vi "Analyze GB - Detail.vi"(8 "Integer Tolerance":dbl=0.1, 10 "Find Integer Rep?":bool, 11 "Grain Boundary Definition":T1={"Grain 1 Orientation"=[1.0, 1.0, 1.0], "Grain 2 Orientation"=[1.0, 1.0, 1.0], "Twist Angle (Deg)"=60.0, "Translation Vector"=[0.0, 0.0, 0.0]}) -> (0 "STEM Viewing Angles":dbl[][](array[numeric]), 1 "Misorientation":T3={"Misorientation Angle"=0.0, "Misorientation Axis, o"=[1.0, 1.0, 1.0], "Misorientation Matrix"=[]}, 2 "Grain 2 Integers":dbl[](array[numeric])=[1.0, 1.0, 1.0], 3 "Grain 1 Integers":dbl[](array[numeric])=[1.0, 1.0, 1.0], 4 "Tilt Angle (Deg)":dbl, 5 "Suggested view direction":dbl[](array[numeric])=[1.0, 1.0, 1.0], 6 "GB Name":string, 7 "STEM Viewable?":bool)   [LabVIEW 2010]
uses:
  <vilib>/Analysis/Matrix/Datatypes/RealMatrix.ctl
  <vilib>/Analysis/baseanly.llb/Real A x B.vi
  <vilib>/Analysis/_algsub.llb/Real Matrix Trace.vi
  <vilib>/Analysis/NI_AALPro.lvlib
  <vilib>/Analysis/NI_AALBase.lvlib
  <vilib>/Analysis/Matrix/NI_Matrix.lvlib
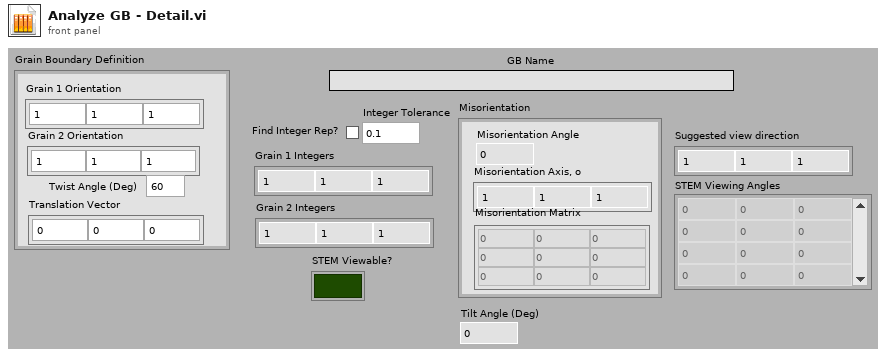
[diagram p1: front panel]
types:
  T1 = cluster{"Grain 1 Orientation":dbl[], "Grain 2 Orientation":dbl[], "Twist Angle (Deg)":dbl, "Translation Vector":dbl[]}
  T2 = typedef "NI_Matrix.lvlib/RealMatrix.ctl" = dbl[][]
  T3 = cluster{"Misorientation Angle":dbl, "Misorientation Axis, o":dbl[], "Misorientation Matrix":T2}
  T4 = cluster{"Grain 1 Orientation":dbl[], "Grain 2 Orientation":dbl[], "Twist Angle (Deg)":dbl}
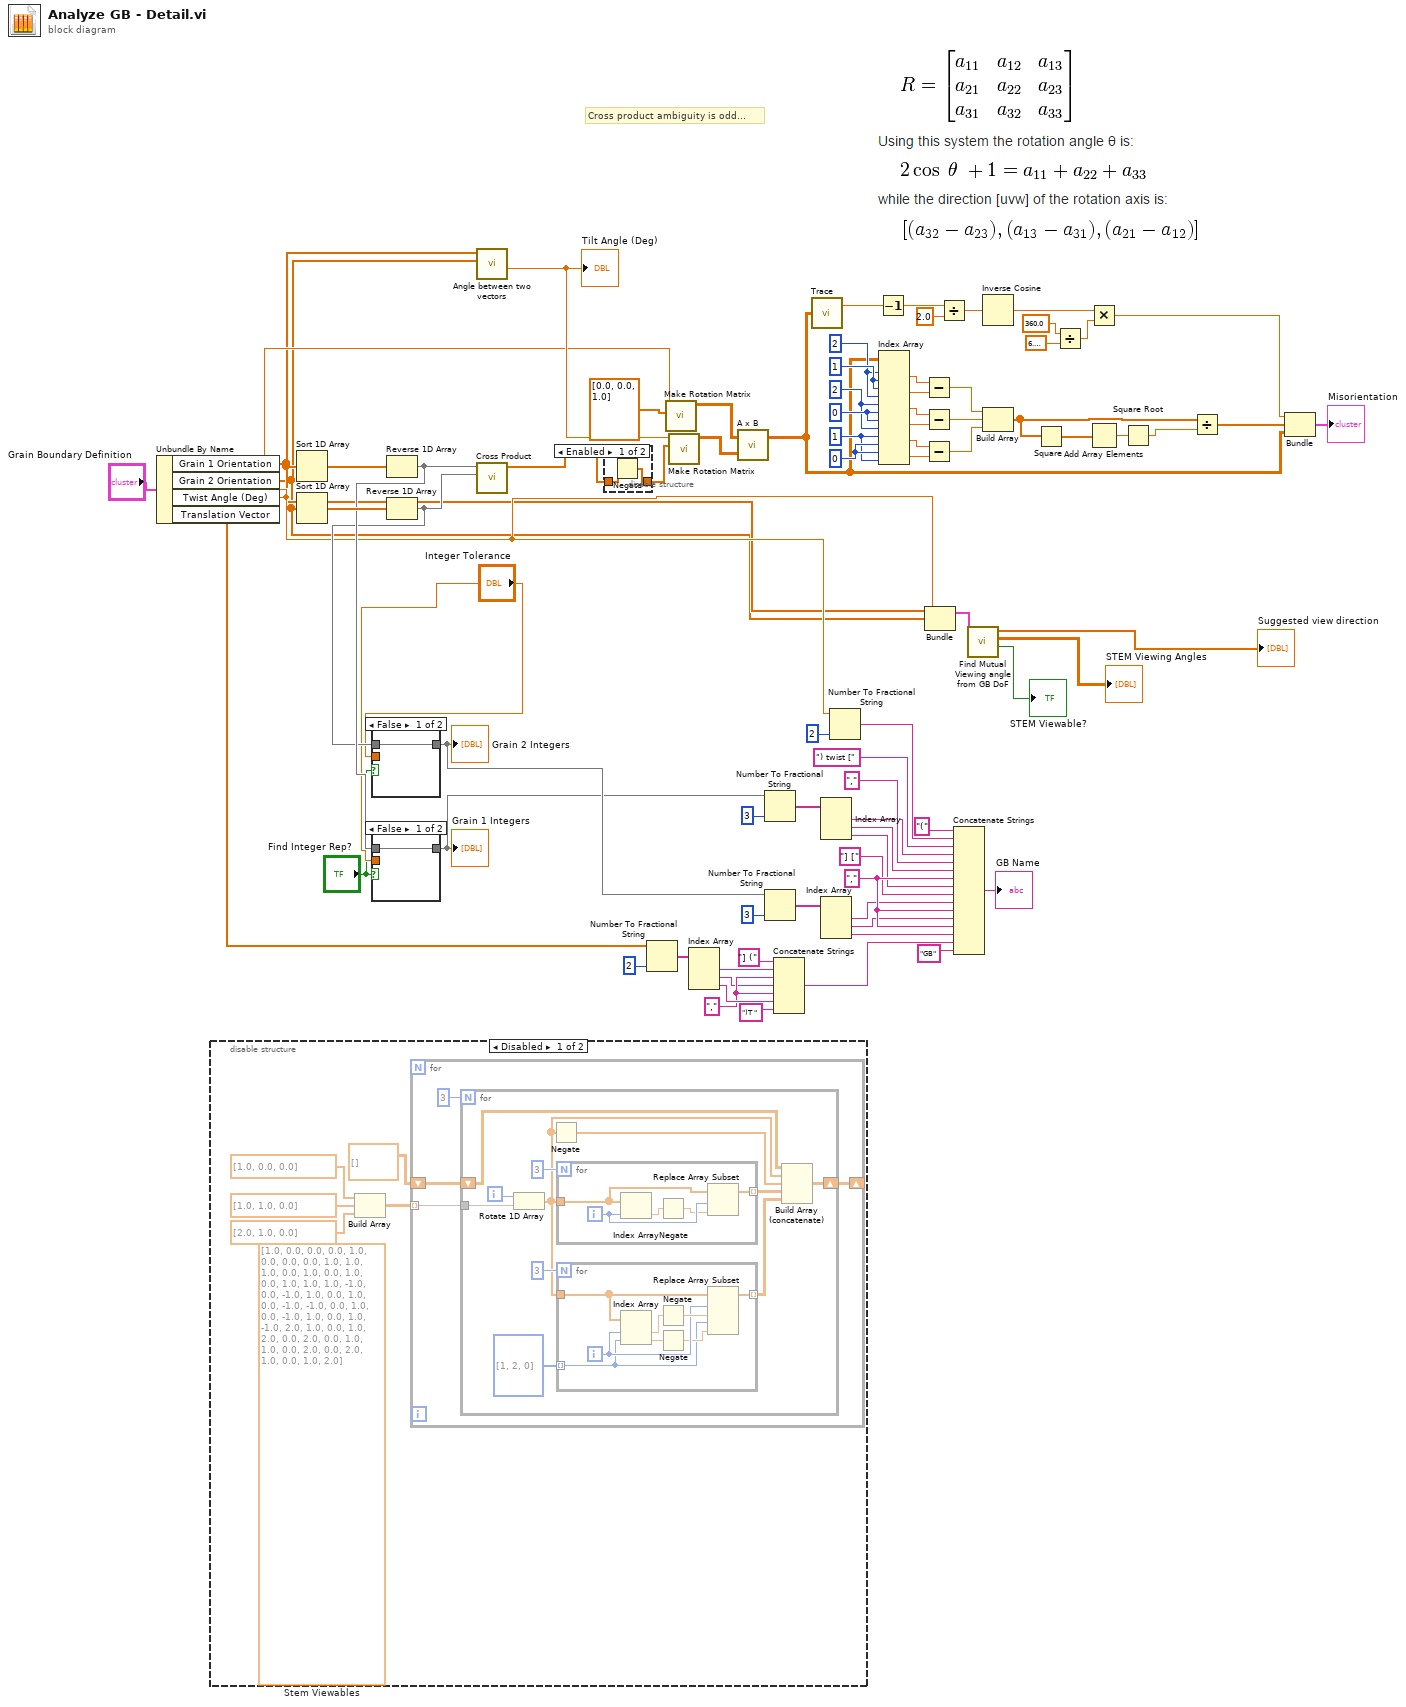
[diagram p0: block diagram]
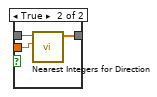
[diagram p3: hidden frame]
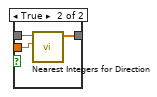
[diagram p4: hidden frame]
diagram:
  w38 = "," ("string")
  w31 = "," ("string")
  w63 = 0 ("index (row)")
  w62 = 1 ("index (row)")
  w65 = 0 ("disabled index (col)")
  w64 = 2 ("index (row)")
  w67 = 1 ("disabled index (col)")
  w66 = 2 ("index (row)")
  # "Cross product ambiguity is odd..."
  n1 = Unbundle By Name("Grain Boundary Definition") -> ("Grain 1 Orientation"=w3:dbl[], "Grain 2 Orientation"=w2:dbl[], "Twist Angle (Deg)"=w8:dbl, "Translation Vector"=w9:dbl[])
  n2 = disable-structure shown="Disabled" {
    frame Disabled {
      (unwired) dbl[][] [[1.0, 0.0, 0.0], [0.0, 1.0, 0.0], [0.0, 0.0, 1.0], [1.0, 1.0, 0.0], [1.0, 0.0, 1.0], [0.0, 1.0, 1.0], [1.0, -1.0, 0.0], [-1.0, 1.0, 0.0], [1.0, 0.0, -1.0], [-1.0, 0.0, 1.0], [0.0, -1.0, 1.0], [0.0, 1.0, -1.0], [2.0, 1.0, 0.0], [1.0, 2.0, 0.0], [2.0, 0.0, 1.0], [1.0, 0.0, 2.0], [0.0, 2.0, 1.0], [0.0, 1.0, 2.0]]  # Stem Viewables
      n3 = Build Array(dbl[] [1.0, 0.0, 0.0] ("Grain 1 Orientation 2"), dbl[] [1.0, 1.0, 0.0] ("Grain 1 Orientation 2"), dbl[] [2.0, 1.0, 0.0] ("Grain 1 Orientation 2")) -> (w84:dbl[][])
      n4 = for {
        tunnel: w84 -> [w90] mode=indexing
        shift-right: [w89] -> _
        shift-left: dbl[][] [] -> [w88]
        n5 = for {
          N: 3 -> [_]
          tunnel: w90 -> [w102]
          shift-right: [w96] -> w89
          shift-left: w88 -> [w95]
          i -> [w101]
          n6 = Rotate 1D Array(1:w102, 2:w101) -> (0:w92:dbl[])
          n7 = Negate(x=w92) -> (-x=w93:dbl[])
          n8 = for {
            N: 3 -> [_]
            tunnel: w92 -> [w114]
            tunnel: [w111] -> w98 mode=indexing
            i -> [w113]
            n9 = Index Array(array=w114, index=w113) -> (element=w115:dbl)
            n10 = Negate(x=w115) -> (-x=w112:dbl)
            n11 = Replace Array Subset(array=w114, new element=w112, index=w113) -> (w111:dbl[])
          }
          n12 = for {
            N: 3 -> [_]
            tunnel: w92 -> [w109]
            tunnel: [w106] -> w97 mode=indexing
            tunnel: i32[] [1, 2, 0] -> [w103] mode=indexing
            i -> [w105]
            n13 = Index Array(array=w109, index #1=w105, index #2=w103) -> (element #1=w110:dbl, element #2=w107:dbl)
            n14 = Negate(x=w110) -> (-x=w108:dbl)
            n15 = Negate(x=w107) -> (-x=w104:dbl)
            n16 = Replace Array Subset(array=w109, new element #1=w108, index #1=w105, new element #2=w104, index #2=w103) -> (w106:dbl[])
          }
          n17 = Build Array (concatenate)(w95, w92, w93, w98, w97) -> (w96:dbl[][])
        }
      }
    }
    frame Enabled {
    }
  }
  n18 = Sort 1D Array(array=w3) -> (sorted array=w82:dbl[])
  n19 = Sort 1D Array(array=w2) -> (sorted array=w81:dbl[])
  n20 = Reverse 1D Array(array=w82) -> (reversed array=w56:dbl[])
  n21 = case shown="False" "Find Integer Rep?" {
    tunnel: [w116 w119] -> w10
    tunnel: w56 -> [w116 w118]
    tunnel: "Integer Tolerance" -> [_ w117]
    frame False {
    }
    frame True {
      n22 = call "Nearest Integers for Direction.vi"("Tolerance"=w117, "Direction"=w118) -> ("Nearest Integer Directions"=w119:dbl[])  [unwired: 8 in, 1 out]
    }
  }
  "Grain 1 Integers" <- w10
  n23 = Reverse 1D Array(array=w81) -> (reversed array=w51:dbl[])
  n24 = case shown="False" "Find Integer Rep?" {
    tunnel: [w120 w123] -> w11
    tunnel: w51 -> [w120 w122]
    tunnel: "Integer Tolerance" -> [_ w121]
    frame False {
    }
    frame True {
      n25 = call "Nearest Integers for Direction.vi"("Tolerance"=w121, "Direction"=w122) -> ("Nearest Integer Directions"=w123:dbl[])  [unwired: 8 in, 1 out]
    }
  }
  "Grain 2 Integers" <- w11
  n26 = call "Angle between two vectors.vi"("Vector 2"=w2, "Vector 1"=w3) -> ("Angle (Degrees)"=w72:dbl)  [unwired: 7 in, 2 out]
  "Tilt Angle (Deg)" <- w72
  n27 = call <vilib>:"Cross Product.vi"("B Vector"=w51, "A Vector"=w56) -> ("Cross Product"=w43:dbl[])  [unwired: 8 in, 1 out]
  n28 = disable-structure shown="Enabled" {
    disable-tunnel: w43 -> [w125 w126]
    disable-tunnel: [w124 w126] -> w42
    frame Enabled {
      n29 = Negate(x=w125) -> (-x=w124:dbl[])
    }
    frame Disabled {
    }
  }
  n30 = Number To Fractional String(number=w9, precision (6)=i16 2) -> (F-format string=w34:string[])  [unwired: 2 in]
  n31 = call "Make Rotation Matrix.vi"("Rotation Axis"=dbl[] [0.0, 0.0, 1.0], "Rotation Angle (Degree)"=w8) -> ("Rotation Matrix"=w44:T2)  [unwired: 9 in]
  n32 = call "Make Rotation Matrix.vi"("Rotation Axis"=w42, "Rotation Angle (Degree)"=w72) -> ("Rotation Matrix"=w45:T2)  [unwired: 9 in]
  n33 = Index Array(array=w34) -> (element #1=w35:string, element #2=w37:string, element #3=w39:string)  [unwired: 3 in]
  n34 = call-poly <vilib>:"A x B.vi"("B"=w45, "A"=w44) -> ("A x B"=w47:T2)  [unwired: 1 out]
  n35 = Number To Fractional String(number=w10, precision (6)=i16 3) -> (F-format string=w18:string[])  [unwired: 2 in]
  n36 = Number To Fractional String(number=w11, precision (6)=i16 3) -> (F-format string=w16:string[])  [unwired: 2 in]
  n37 = Concatenate Strings("] (" ("string"), w35, w38, w37, w38, w39, ")T " ("string")) -> (w15:string)
  n38 = call-poly <vilib>:"Trace.vi"("Input Matrix"=w47) -> ("trace"=w80:dbl)  [unwired: 1 out]
  n39 = Index Array(array=w18) -> (element #1=w24:string, element #2=w26:string, element #3=w27:string)  [unwired: 3 in]
  n40 = Index Array(array=w16) -> (element #1=w29:string, element #2=w30:string, element #3=w32:string)  [unwired: 3 in]
  n41 = Number To Fractional String(number=w8, precision (6)=i16 2) -> (F-format string=w22:string)  [unwired: 2 in]
  n42 = Decrement(x=w80) -> (x-1=w79:dbl)
  n43 = Index Array(array=w47, index (row) #1=w66, index (col) #1=w67, index (row) #2=w67, index (col) #2=w66, index (row) #3=w64, index (col) #3=w65, index (row) #4=w65, index (col) #4=w64, index (row) #5=w62, index (col) #5=w63, index (row) #6=w63, index (col) #6=w62) -> (element #1=w71:dbl, element #2=w70:dbl, element #3=w69:dbl, element #4=w68:dbl, element #5=w61:dbl, element #6=w60:dbl)
  n44 = Subtract(x=w71, y=w70) -> (x-y=w59:dbl)
  n45 = Subtract(x=w69, y=w68) -> (x-y=w58:dbl)
  n46 = Subtract(x=w61, y=w60) -> (x-y=w57:dbl)
  n47 = Bundle("Grain 1 Orientation"=w3, "Grain 2 Orientation"=w2, "Twist Angle (Deg)"=w8) -> (w7:T4)  [unwired: 1 in]
  n48 = Divide(x=w79, y=2.0) -> (x/y=w77:dbl)
  n49 = Concatenate Strings("(" ("string"), w22, ") twist [" ("string"), w24, "," ("string"), w26, w31, w27, "] [" ("string"), w29, w31, w30, w31, w32, w15, "GB" ("string")) -> (→"GB Name":string)
  n50 = call "Find Mutual Viewing angle from GB DoF.vi"("Grain Boundary Macro DoF"=w7) -> ("STEM Viewable?"=→"STEM Viewable?":bool, "STEM Viewing Angles"=→"STEM Viewing Angles":dbl[][], "Mutual Viewing Angle"=→"Suggested view direction":dbl[])  [unwired: 8 in]
  n51 = Inverse Cosine(1:w77) -> (0:w73:dbl)
  n52 = Build Array(w59, w58, w57) -> (w52:dbl[])
  n53 = Square(x=w52) -> (x^2=w53:dbl[])
  n54 = Divide(x=360.0, y=6.283185307179586) -> (x/y=w76:dbl)
  n55 = Multiply(x=w73, y=w76) -> (x*y=w49:dbl)
  n56 = Add Array Elements(numeric array=w53) -> (sum=w54:dbl)
  n57 = Square Root(x=w54) -> (sqrt(x)=w55:dbl)
  n58 = Divide(x=w52, y=w55) -> (x/y=w48:dbl[])
  n59 = Bundle(w49, w48, "A x B"=w47) -> (→"Misorientation":cluster{dbl, dbl[], "A x B":T2})  [unwired: 1 in]
